vi "Drive Controller.vi"(8 "error in":errorcluster) -> ()   [LabVIEW 2015]
doc: "This VI executes continuously carrying out the current operation and responding to updates or new operation requests. It will often contain the timing or control code that is difficult to place directly in TeleOp. This VI generally opens all sensors and motors and isolates the rest of the robot code from knowing implementation details of how the operations are carried out."
uses:
  Drive Setpoints.ctl
  Drive Operations.ctl
  <vilib>/Rock Robotics/WPI/SafetyOutput/WPI_SafetyOutputConfigMenu.ctl
  <vilib>/Rock Robotics/WPI/CAN/TalonSRX/WPI_CANTalonSRX_APIControlMode.ctl
  JoystickData.ctl
  <vilib>/Rock Robotics/WPI/Utilities/WPI_GetSetVariantRefNum.vi
  Global Drive Variables.vi
panel:
  in  "Numeric":dbl
  out "Setpoints":T1(graph)
  out "Current\nCmd":string
  # "Tip: It may be helpful to observe inputs and sensor values.\nYou may also want to display tuning or debugging controls."
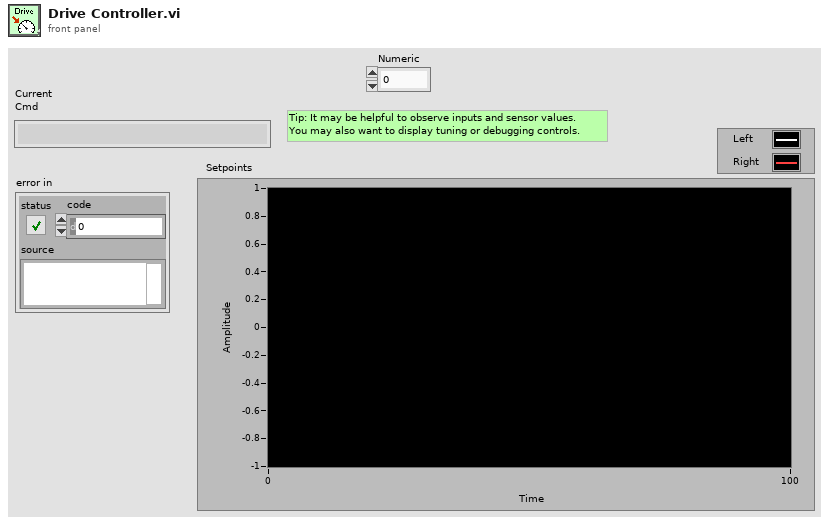
[diagram p1: front panel]
types:
  T1 = cluster{"Left Setpoint":dbl, "Right Setpoint":dbl}
  T2 = typedef "WPI_CANTalonSRX_APIControlMode.ctl" = enum8{"Percent VBus", "Speed", "Position", "Slave", "Unchanged / Invalid", "Voltage Compensation", "Current", "Motion Profile"}
  T3 = typedef "WPI_SafetyOutputConfigMenu.ctl" = enum16{"Enable", "Disable"}
  T4 = typedef "Drive Setpoints.ctl" = cluster{"Operation":T5, "Left Setpoint":dbl, "Right Setpoint":dbl, "Duration":dbl}
  T5 = typedef "Drive Operations.ctl" = enum16{"Reserve", "Read Current", "Immediate", "Drive for Time", "Drive for Distance"}
  T6 = typedef "WPI_MotorControlDeviceRef.ctl" = cluster{"DeviceStatus":errorcluster, "Type":T7, "PWM":cluster{"PWM Channel":T8, "DeadBand":T9}, "CAN":cluster{"Device Number":u8, "Control Mode":T10, "Semaphore":T11, "Max Vout":dbl, "TalonSRX Control Mode":T2}, "Invert":bool}
  T7 = typedef "WPI_MotorControlType.ctl" = enum16{"PWM", "CAN", "CANTalonSRX"}
  T8 = typedef "FPGA_DIOPWMChannel.ctl" = enum8{"PWM 0", "PWM 1", "PWM 2", "PWM 3", "PWM 4", "PWM 5", "PWM 6", "PWM 7", "PWM 8", "PWM 9", "PWM MXP 0", "PWM MXP 1", "PWM MXP 2", "PWM MXP 3", "PWM MXP 4", "PWM MXP 5", "PWM MXP 6", "PWM MXP 7", "PWM MXP 8", "PWM MXP 9", "Invalid"}
  T9 = typedef "WPI_PWMDeadband.ctl" = cluster{"Name":string, "maxPositivePwm":i32, "minPositivePwm":i32, "centerPwm":i32, "maxNegativePwm":i32, "minNegativePwm":i32, "angularRange":u16}
  T10 = typedef "WPI_CANJaguar_ControlMode.ctl" = enum8{"Percent VBus", "Current", "Speed", "Position", "Voltage"}
  T11 = typedef "Semaphore RefNum" = refnum<k1>
  T12 = typedef "WPI_RobotDriveDevRef.ctl" = cluster{"DevStatus":errorcluster, "Motors[]":T6[], "Square Inputs":bool, "Max Output":dbl}
  T13 = typedef "Command Status Info.ctl" = cluster{"Name":string, "Status":T14, "notifier out":T15}
  T14 = typedef "Completion Status.ctl" = enum16{"Successful", "Aborted", "Incomplete"}
  T15 = typedef "Completion Notifier.ctl" = refnum<notifier>
  T16 = cluster{"SubSystem Data":T4, cluster{"Start Time (ms)":u32, "Iterations":i32}, cluster{"Command Info":T13, "Description":string, "SubSystem Data":T4, "notifier out":refnum<notifier>, "Subsystem Name":string}}
  T17 = cluster{"SubSystem Data":T4, cluster{"Start Time (ms)":u32, "Iterations":i32}, "Default Command Arguments":cluster{"Command Info":T13, "Description":string, "SubSystem Data":T4, "notifier out":refnum<notifier>, "Subsystem Name":string}}
  T18 = cluster{"Don't move motors while reserved":dbl, "Don't move motors while reserved":dbl}
  T19 = typedef "JoystickData.ctl" = cluster{"Axes":dbl[], "Buttons":bool[]}
  T20 = typedef "WPI_JoystickDevRef.ctl" = cluster{"Device":T21}
  T21 = typedef "WPI_JoystickDeviceEnum.ctl" = enum16{"USB 0", "USB 1", "USB 2", "USB 3", "USB 4", "USB 5"}
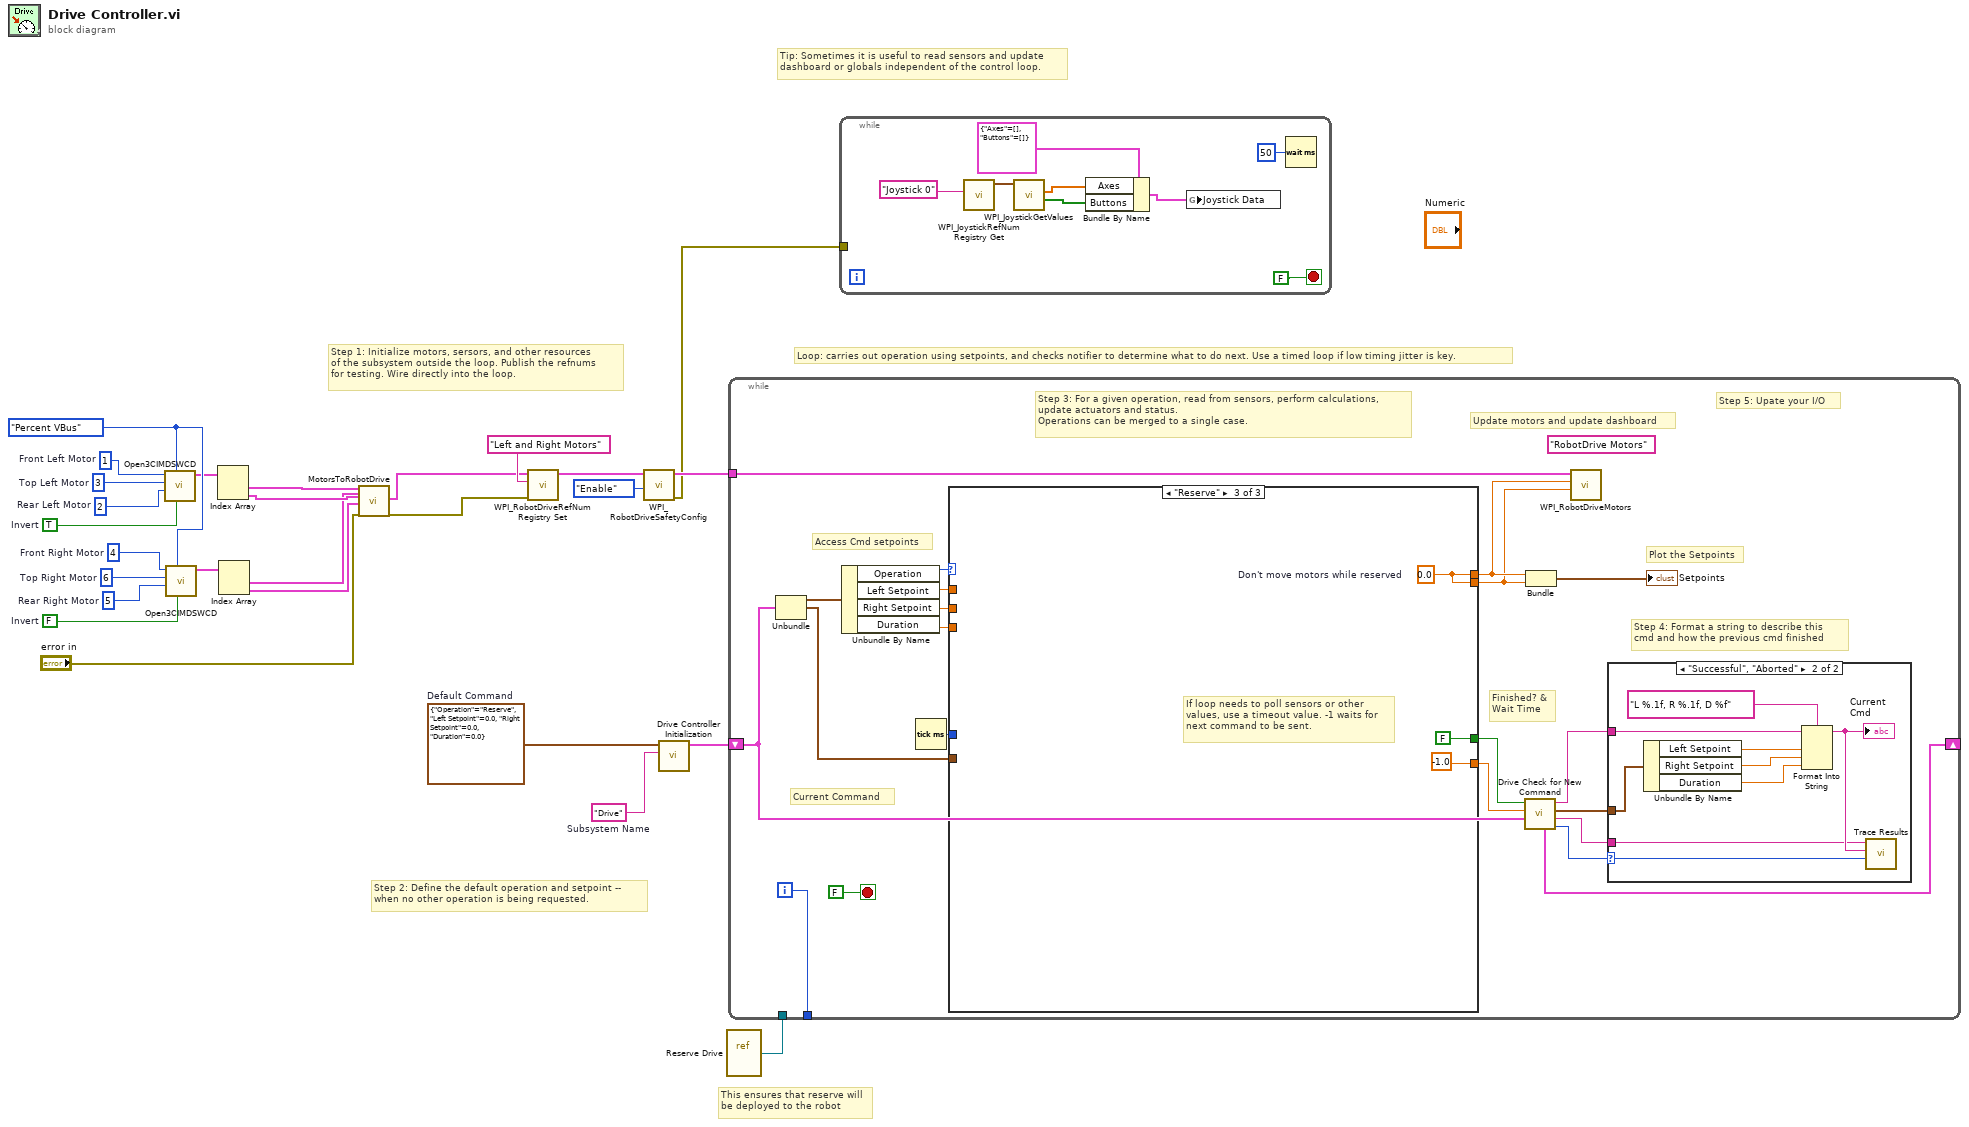
[diagram p0: block diagram]
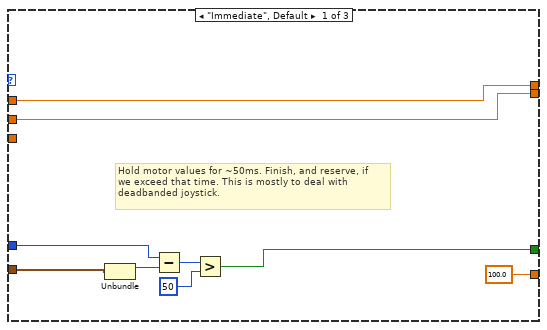
[diagram p3: hidden frame]
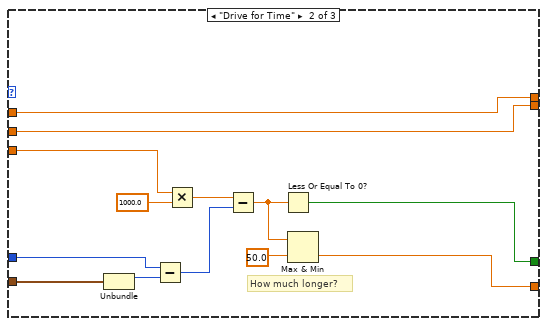
[diagram p4: hidden frame]
diagram:
  w11 = FALSE  # Invert
  w16 = TRUE  # Invert
  w13 = u8 6  # Top Right Motor
  w12 = u8 5  # Rear Right Motor
  w14 = u8 4  # Front Right Motor
  w18 = u8 3  # Top Left Motor
  w17 = u8 2  # Rear Left Motor
  w19 = u8 1  # Front Left Motor
  w15 = WPI_CANTalonSRX_APIControlMode."Percent VBus" ("Control Mode")
  w26 = T4 {"Operation"=enum."Reserve", "Left Setpoint"=0.0, "Right Setpoint"=0.0, "Duration"=0.0}  # Default Command
  w27 = "Drive"  # Subsystem Name
  # "This ensures that reserve will\nbe deployed to the robot"
  # "Tip: Sometimes it is useful to read sensors and update\ndashboard or globals independent of the control loop."
  # "Step 2: Define the default operation and setpoint --\nwhen no other operation is being requested."
  # "Step 1: Initialize motors, sersors, and other resources\nof the subsystem outside the loop. Publish the refnums\nfor testing. Wire directly into the loop."
  # "Loop: carries out operation using setpoints, and checks notifier to determine what to do next. Use a timed loop if low timing jitter is key."
  n1 = call "Open3CIMDSWCD.vi"("Invert"=w16, "Control Mode"=w15, "Bottom Back"=w17, "Top Middle"=w18, "Bottom Front"=w19) -> ("Motor Instances"=w10:T6[])  [unwired: 6 in]
  n2 = call "Open3CIMDSWCD.vi"("Invert"=w11, "Control Mode"=w15, "Bottom Back"=w12, "Top Middle"=w13, "Bottom Front"=w14) -> ("Motor Instances"=w7:T6[])  [unwired: 6 in]
  n3 = Index Array(array=w10) -> (element #1=w9:T6, element #2=w8:T6)  [unwired: 2 in]
  n4 = Index Array(array=w7) -> (element #1=w6:T6, element #2=w5:T6)  [unwired: 2 in]
  n5 = call "MotorsToRobotDrive.vi"("Left"=w9, "Left 2"=w6, "Right"=w8, "Right 2"=w5, "error in"="error in") -> ("RobotDriveDevRef"=w4:T12, "error out"=w3:errorcluster)  [unwired: 13 in]
  n6 = call <vilib>:"WPI_RobotDriveRefNum Registry Set.vi"("error in (no error)"=w3, "refnum name"="Left and Right Motors", "RobotDriveDevRef"=w4) -> ("RobotDriveDevRef"=w24:T12)  [unwired: 1 in, 7 out]
  n7 = call <vilib>:"WPI_RobotDriveSafetyConfig.vi"("mode"=WPI_SafetyOutputConfigMenu."Enable", "RobotDriveDevRef"=w24) -> ("error out"=w1:errorcluster, "RobotDriveDevRef"=w22:T12)  [unwired: 8 in]
  n8 = call "Drive Controller Initialization.vi"("Subsystem Name"=w27, "Default Command"=w26) -> ("output cluster"=w21:T16)  [unwired: 9 in]
  n9 = vi-ref "Reserve Drive.vi"() -> (w20:refnum<vi>)
  n10 = while {
    shift-right: [w35] -> _
    shift-left: w21 -> [w28]
    tunnel: [w47] -> _
    tunnel: w22 -> [w43]
    tunnel: w20 -> [_]
    i -> [w47]
    stop <- FALSE stop-if-true
    (unwired) "RobotDrive Motors" ("Name")
    # "Step 5: Upate your I/O"
    # "Step 4: Format a string to describe this\ncmd and how the previous cmd finished"
    # "Current Command"
    # "Update motors and update dashboard"
    # "Plot the Setpoints"
    # "Access Cmd setpoints"
    # "Finished? &\nWait Time"
    # "Step 3: For a given operation, read from sensors, perform calculations,\nupdate actuators and status.\nOperations can be merged to a single case."
    n11 = Unbundle(w28) -> ("SubSystem Data"=w42:T4, w29:cluster{"Start Time (ms)":u32, "Iterations":i32})  [unwired: 1 out]
    n12 = Unbundle By Name(w42) -> ("Operation"=w41:T5, "Left Setpoint"=w40:dbl, "Right Setpoint"=w39:dbl, "Duration"=w38:dbl)
    n13 = Tick Count (ms)() -> (millisecond timer value=w37:u32)
    n14 = case shown="\"Reserve\"" w41 {
      tunnel: [100.0 w67 -1.0] -> w34
      tunnel: [w59 w74 FALSE ("ignore previous (F)")] -> w33
      tunnel: w29 -> [w58 w76 _]
      tunnel: [w65 w73 w80] -> w45
      tunnel: [w64 w72 w80] -> w44
      tunnel: w40 -> [w65 w73 _]
      tunnel: w39 -> [w64 w72 _]
      tunnel: w38 -> [_ w71 _]
      tunnel: w37 -> [w60 w70 _]
      frame "Immediate", Default {
        # "Hold motor values for ~50ms. Finish, and reserve, if\nwe exceed that time. This is mostly to deal with\ndeadbanded joystick."
        n15 = Unbundle(w58) -> ("Start Time (ms)"=w61:u32)  [unwired: 1 out]
        n16 = Subtract(x=w60, y=w61) -> (x-y=w62:u32)
        n17 = Greater?(x=w62, y=u8 50 ("Left Motor")) -> (0:w59:bool)
      }
      frame "Drive for Time" {
        # "How much longer?"
        n18 = Unbundle(w76) -> ("Start Time (ms)"=w75:u32)  [unwired: 1 out]
        n19 = Subtract(x=w70, y=w75) -> (x-y=w79:u32)
        n20 = Multiply(x=w71, y=1000.0) -> (x*y=w78:dbl)
        n21 = Subtract(x=w78, y=w79) -> (x-y=w69:dbl)
        n22 = Less Or Equal To 0?(x=w69) -> (x <= 0?=w74:bool)
        n23 = Max & Min(x=w69, y=50.0) -> (min(x,y)=w67:dbl)  [unwired: 1 out]
      }
      frame "Reserve" {
        w80 = 0.0  # Don't move motors while reserved
        # "If loop needs to poll sensors or other\nvalues, use a timeout value. -1 waits for\nnext command to be sent."
      }
    }
    n24 = call "Drive Check for New Command.vi"("input cluster"=w28, "Wait time (ms)"=w34, "Finished?"=w33) -> ("Completion"=w36:T14, "Subsystem Name"=w30:string, "SetPoint"=w31:T4, "Initial Trace String"=w32:string, "output cluster"=w35:T17)  [unwired: 4 in]
    n25 = Bundle("Don't move motors while reserved"=w45, "Don't move motors while reserved"=w44) -> (→"Setpoints":T18)  [unwired: 1 in]
    n26 = call <vilib>:"WPI_RobotDriveMotors.vi"("RightSpeed"=w44, "LeftSpeed"=w45, "RobotDriveDevRef"=w43) -> ()  [unwired: 1 in, 8 out]
    n27 = case shown="\"Successful\", \"Aborted\"" w36 {
      selector: w36 -> [_ w57]
      tunnel: w32 -> [_ w52]
      tunnel: w31 -> [_ w53]
      tunnel: w30 -> [_ w49]
      frame "Incomplete", Default {
        # "Continuing current command"
      }
      frame "Successful", "Aborted" {
        # "Report and setup for next command"
        n28 = Unbundle By Name(w53) -> ("Left Setpoint"=w55:dbl, "Right Setpoint"=w56:dbl, "Duration"=w50:dbl)
        n29 = Format Into String(format string="L %.1f, R %.1f, D %f", initial string=w52, w55, w56, w50) -> (resulting string=w51:string)  [unwired: 1 in, 1 out]
        "Current\nCmd" <- w51
        n30 = call <vilib>:"Trace Results.vi"("Status of previous command"=w57, "Description"=w51, "Subsystem"=w49) -> ()  [unwired: 9 in]
      }
    }
  }
  n31 = while {
    tunnel: w1 -> [_]
    stop <- FALSE stop-if-true
    n32 = call <vilib>:"WPI_JoystickRefNum Registry Get.vi"("refnum name"="Joystick 0") -> ("JoystickDevRef"=w88:T20)  [unwired: 1 in, 9 out]
    n33 = call <vilib>:"WPI_JoystickGetValues.vi"("JoystickDevRef"=w88) -> ("Buttons"=w83:bool[], "Axes"=w84:dbl[])  [unwired: 6 in, 3 out]
    n34 = Bundle By Name(cluster=T19 {"Axes"=[], "Buttons"=[]} ("Joystick Data"), "Axes"=w84, "Buttons"=w83) -> (w86:T19)
    n35 = global write "Global Drive Variables.vi" "Joystick Data"(w86) -> ()
    n36 = Wait (ms)(milliseconds to wait=u32 50) -> ()  [unwired: 1 out]
  }
